vi "MicrometerDiff.vi"() -> ()   [LabVIEW 2015]
uses:
  <vilib>/Analysis/baseanly.llb/Mean (DBL).vi
  <vilib>/Utility/file.llb/Read From Spreadsheet File (DBL).vi
  <vilib>/Analysis/NI_AALBase.lvlib
panel:
  in  "200,1100":dbl format="%.2g"
  in  "800,1100":dbl format="%.2g"
  in  "1200, 1100":dbl format="%.2g"
  in  "1550,1100":dbl format="%.2g"
  in  "2000,1100":dbl format="%.2g"
  in  "2200,400":dbl format="%.2g"
  in  "2200,500":dbl format="%.2g"
  in  "2000,200":dbl format="%.2g"
  in  "1550,200":dbl format="%.2g"
  in  "1200,200":dbl format="%.2g"
  in  "800,200":dbl format="%.2g"
  in  "200,200":dbl format="%.2g"
  in  "0,500":dbl format="%.2g"
  in  "0,400":dbl format="%.2g"
  out "x         y         DR      Meas    Diff(um)":dbl[][](array[numeric]) format="%#_4f"
  out "nome file":string="micrometer_"
  in  "suffisso (se necessario)":string
  out "rms value":dbl format="%0.2f"
  out "mean":dbl format="%0.2f"
  out "appended array":dbl[](array[numeric])
  in  "stop":bool
  # "Micrometer Measurement\n(difference w.r.t. empty Dry Run)"
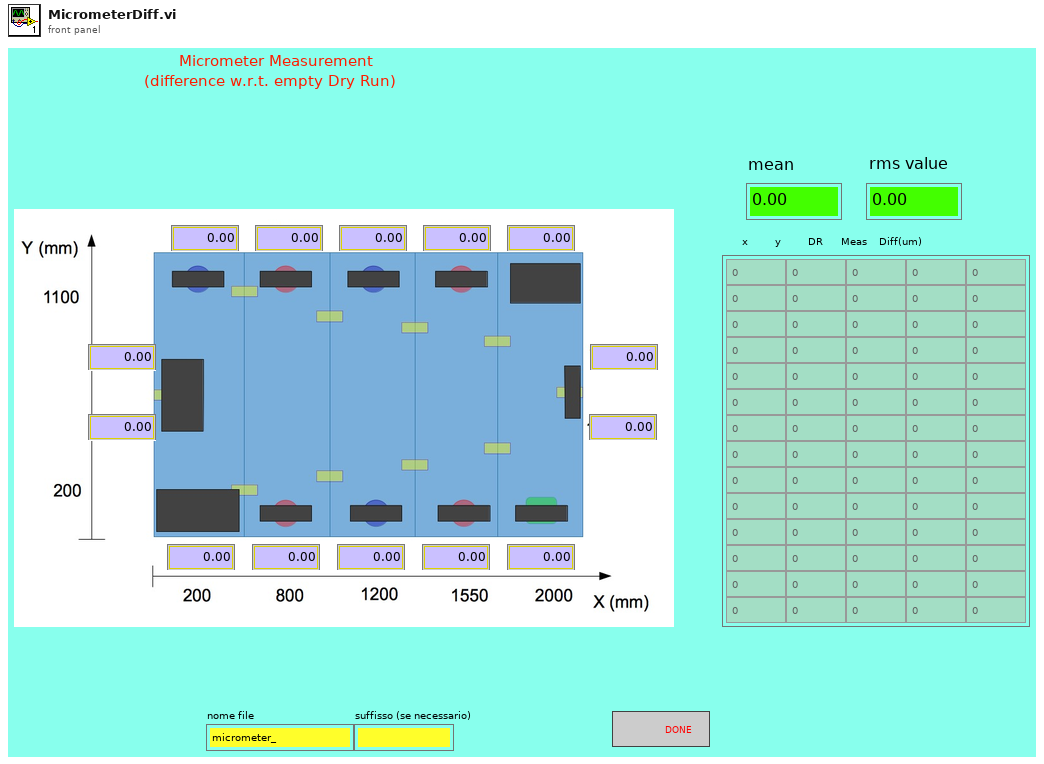
[diagram p1: front panel]
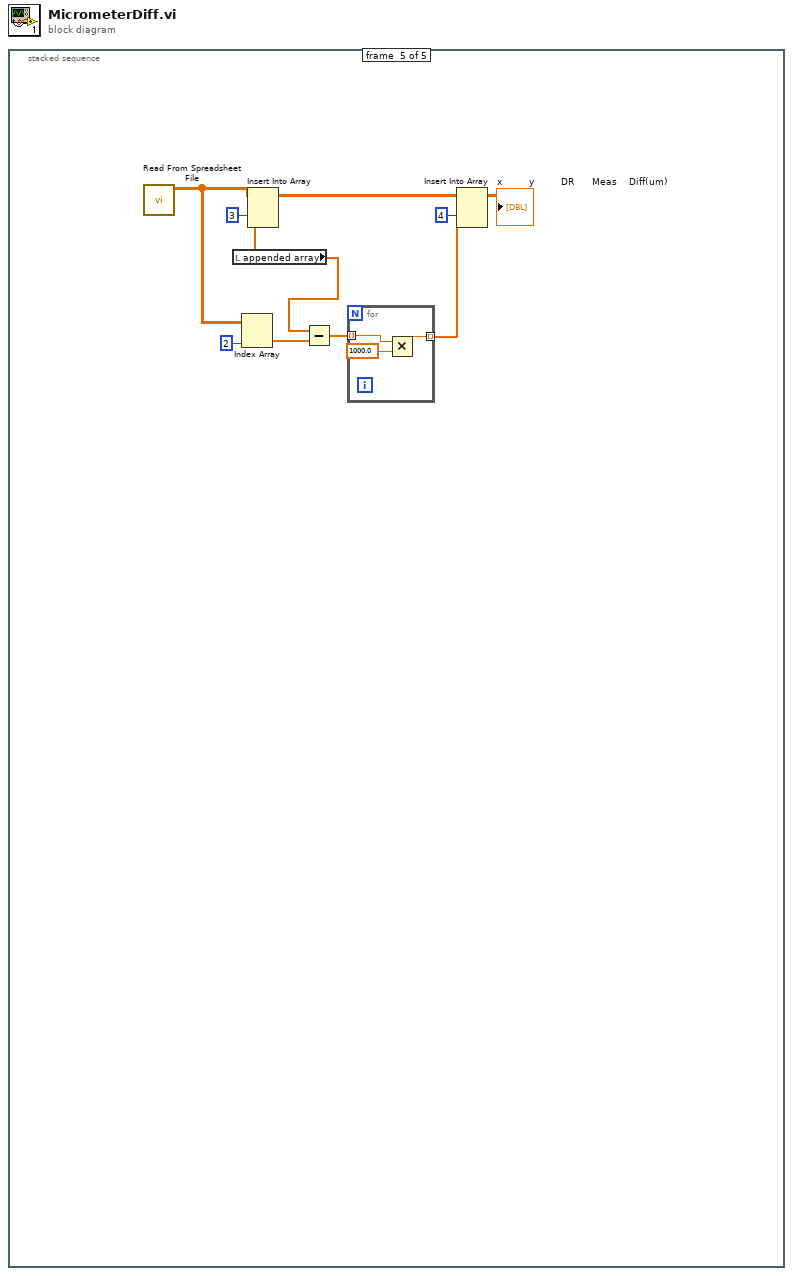
[diagram p0: block diagram]
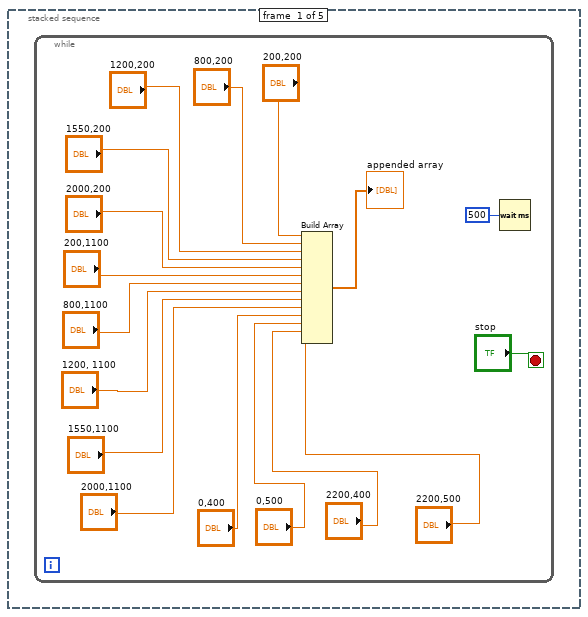
[diagram p2: hidden frame]
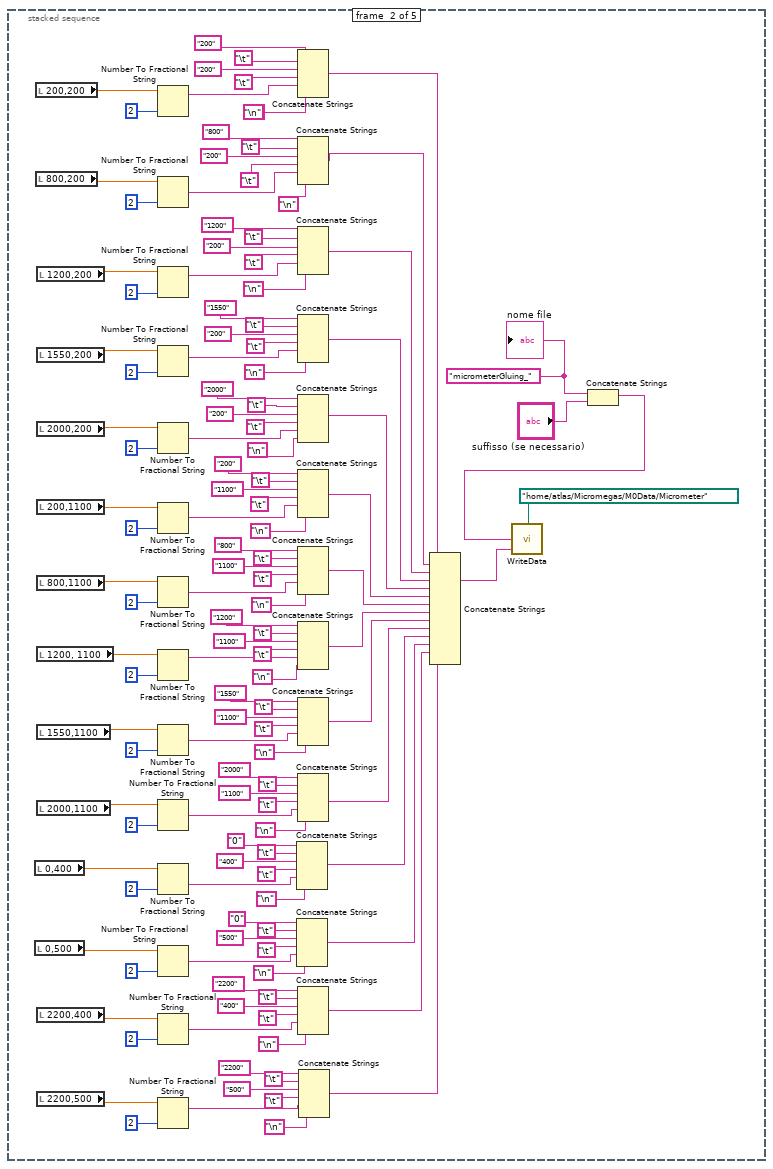
[diagram p3: hidden frame]
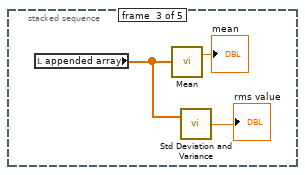
[diagram p4: hidden frame]
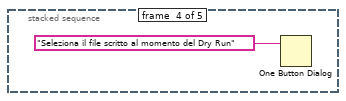
[diagram p5: hidden frame]
diagram:
  n1 = stacked-sequence {
    frame #0 {
      n2 = while {
        stop <- "stop" stop-if-true
        n3 = Build Array("200,200", "800,200", "1200,200", "1550,200", "2000,200", "200,1100", "800,1100", "1200, 1100", "1550,1100", "2000,1100", "0,400", "0,500", "2200,400", "2200,500") -> (→"appended array":dbl[])
        n4 = Wait (ms)(milliseconds to wait=u32 500) -> ()  [unwired: 1 out]
      }
    }
    frame #1 {
      w25 = "micrometerGluing_" ("string")
      (unwired) "\n"
      n5 = local read "0,400"() -> (w19:dbl)
      n6 = local read "0,500"() -> (w18:dbl)
      n7 = local read "200,200"() -> (w20:dbl)
      n8 = local read "800,200"() -> (w21:dbl)
      n9 = local read "1200,200"() -> (w113:dbl)
      n10 = local read "1550,200"() -> (w112:dbl)
      n11 = local read "2000,200"() -> (w111:dbl)
      n12 = local read "200,1100"() -> (w76:dbl)
      n13 = local read "800,1100"() -> (w75:dbl)
      n14 = local read "1200, 1100"() -> (w74:dbl)
      n15 = local read "1550,1100"() -> (w73:dbl)
      n16 = local read "2000,1100"() -> (w72:dbl)
      n17 = local read "2200,400"() -> (w47:dbl)
      n18 = local read "2200,500"() -> (w46:dbl)
      n19 = Number To Fractional String(number=w20, precision (6)=i16 2) -> (F-format string=w143:string)  [unwired: 2 in]
      n20 = Number To Fractional String(number=w21, precision (6)=i16 2) -> (F-format string=w137:string)  [unwired: 2 in]
      n21 = Number To Fractional String(number=w113, precision (6)=i16 2) -> (F-format string=w122:string)  [unwired: 2 in]
      n22 = Number To Fractional String(number=w112, precision (6)=i16 2) -> (F-format string=w128:string)  [unwired: 2 in]
      n23 = Number To Fractional String(number=w111, precision (6)=i16 2) -> (F-format string=w134:string)  [unwired: 2 in]
      n24 = Number To Fractional String(number=w76, precision (6)=i16 2) -> (F-format string=w110:string)  [unwired: 2 in]
      n25 = Number To Fractional String(number=w75, precision (6)=i16 2) -> (F-format string=w103:string)  [unwired: 2 in]
      n26 = Number To Fractional String(number=w74, precision (6)=i16 2) -> (F-format string=w85:string)  [unwired: 2 in]
      n27 = Number To Fractional String(number=w73, precision (6)=i16 2) -> (F-format string=w92:string)  [unwired: 2 in]
      n28 = Number To Fractional String(number=w72, precision (6)=i16 2) -> (F-format string=w82:string)  [unwired: 2 in]
      n29 = Number To Fractional String(number=w19, precision (6)=i16 2) -> (F-format string=w71:string)  [unwired: 2 in]
      n30 = Number To Fractional String(number=w18, precision (6)=i16 2) -> (F-format string=w65:string)  [unwired: 2 in]
      n31 = Number To Fractional String(number=w47, precision (6)=i16 2) -> (F-format string=w53:string)  [unwired: 2 in]
      n32 = Number To Fractional String(number=w46, precision (6)=i16 2) -> (F-format string=w59:string)  [unwired: 2 in]
      n33 = Concatenate Strings("0", "\t", "400", "\t", w71, "\n") -> (w30:string)
      n34 = Concatenate Strings("0", "\t", "500", "\t", w65, "\n") -> (w29:string)
      n35 = Concatenate Strings("200", "\t", "200", "\t", w143, "\n") -> (w40:string)
      n36 = Concatenate Strings("800", "\t", "200", "\t", w137, "\n") -> (w39:string)
      n37 = Concatenate Strings("1200", "\t", "200", "\t", w122, "\n") -> (w38:string)
      n38 = Concatenate Strings("1550", "\t", "200", "\t", w128, "\n") -> (w37:string)
      n39 = Concatenate Strings("2000", "\t", "200", "\t", w134, "\n") -> (w36:string)
      n40 = Concatenate Strings("200", "\t", "1100", "\t", w110, "\n") -> (w35:string)
      n41 = Concatenate Strings("800", "\t", "1100", "\t", w103, "\n") -> (w34:string)
      n42 = Concatenate Strings("1200", "\t", "1100", "\t", w85, "\n") -> (w33:string)
      n43 = Concatenate Strings("1550", "\t", "1100", "\t", w92, "\n") -> (w32:string)
      n44 = Concatenate Strings("2000", "\t", "1100", "\t", w82, "\n") -> (w31:string)
      n45 = Concatenate Strings("2200", "\t", "400", "\t", w53, "\n") -> (w28:string)
      n46 = Concatenate Strings("2200", "\t", "500", "\t", w59, "\n") -> (w27:string)
      n47 = Concatenate Strings(w40, w39, w38, w37, w36, w35, w34, w33, w32, w31, w30, w29, w28, w27) -> (w23:string)
      n48 = Concatenate Strings(w25, "suffisso (se necessario)") -> (w26:string)
      n49 = call "WriteData.vi"("Message"=w23, "File Prefix"=w26, "base path"=path "/home/atlas/Micromegas/M0Data/Micrometer") -> ()
      "nome file" <- w25
    }
    frame #2 {
      n50 = local read "appended array"() -> (w149:dbl[])
      n51 = call-poly <vilib>:"Mean.vi"("X"=w149) -> ("mean"=→"mean":dbl)  [unwired: 1 out]
      n52 = call <vilib>:"Std Deviation and Variance.vi"("X"=w149) -> ("standard deviation"=→"rms value":dbl)  [unwired: 1 in, 2 out]
    }
    frame #3 {
      n53 = One Button Dialog(message="Seleziona il file scritto al momento del Dry Run") -> ()  [unwired: 1 in, 1 out]
    }
    frame #4 {
      n54 = call-poly <vilib>:"Read From Spreadsheet File.vi"() -> ("all rows"=w161:dbl[][])  [unwired: 7 in, 4 out]
      n55 = local read "appended array"() -> (w156:dbl[])
      n56 = Index Array(array=w161, index (col)=2 ("disabled index (col)")) -> (element=w155:dbl[])  [unwired: 1 in]
      n57 = Insert Into Array(array=w161, index (col)=3 ("disabled index (col)"), new element=w156) -> (w159:dbl[][])  [unwired: 1 in]
      n58 = Subtract(x=w156, y=w155) -> (x-y=w154:dbl[])
      n59 = for {
        tunnel: w154 -> [w165] mode=indexing
        tunnel: [w163] -> w153 mode=indexing
        n60 = Multiply(x=w165, y=1000.0) -> (x*y=w163:dbl)
      }
      n61 = Insert Into Array(array=w159, index (col)=4 ("disabled index (col)"), new element=w153) -> (→"x         y         DR      Meas    Diff(um)":dbl[][])  [unwired: 1 in]
    }
  }
